vi "Edit_Server_Channel.vi"(5 "Mode":T1(ring)) -> ()   [LabVIEW 2021]
uses:
  Sub VIs/ADAM Controls/Ch_description_ADAM.ctl
  Sub VIs/ADAM Controls/Module_type_ADAM.ctl
  Sub VIs/ADAM Controls/Function_ADAM.ctl
  Sub VIs/ADAM Controls/Channel_State.ctl
  Sub VIs/ADAM Controls/Calib_type_ADAM.ctl
  Sub VIs/ADAM Controls/Address.ctl
  Sub VIs/ADAM Controls/Channel_names.ctl
panel:
  out "Message":string
  in  "Value":dbl
  out "String":string
  out "Help":string
  in  "Search String":string
  in  "Channel Names":i32(listbox)
  in  "Ch Description":T2={"Ch Name"="", "Type"="", "Function"=enum."Analogue Input", "Ch State"=enum."On", "Calibration type"="", "A"=0.0, "B"=0.0, "C"=0.0, "D"=0.0, "Comments"="", "Address"={"Main"=0, "Ch."=0, "Sub"=0, "Port Name"=""}, "String"="", "Duty"=65535} {"Duty" format="%016b"; "D" format="%#_5g"; "C" format="%#_5g"; "B" format="%#_5g"; "A" format="%#_5g"}
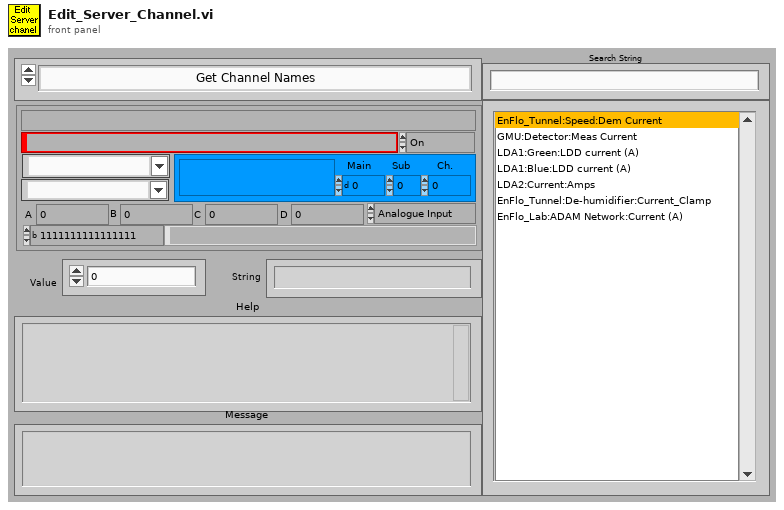
[diagram p1: front panel]
types:
  T1 = enum16{"Get Channel Names", "Get Current Value", "Update Channel Value", "Update Channel Description"}
  T2 = typedef "Ch_description_ADAM.ctl" = cluster{"Ch Name":string, "Type":T3, "Function":T4, "Ch State":T5, "Calibration type":T6, "A":dbl, "B":dbl, "C":dbl, "D":dbl, "Comments":string, "Address":T7, "String":string, "Duty":u16}
  T3 = typedef "Module_type_ADAM.ctl" = string
  T4 = typedef "Function_ADAM.ctl" = enum16{"Analogue Input", "Digital Input", "Event counter", "Event rate", "Analogue Output", "Digital Output", "Relay Output"}
  T5 = typedef "Channel_State.ctl" = enum16{"On", "Off", "Always On", "Always Off"}
  T6 = typedef "Calib_type_ADAM.ctl" = string
  T7 = typedef "Address.ctl" = cluster{"Main":i32, "Ch.":i32, "Sub":i32, "Port Name":string}
  T8 = typedef "Channel_names.ctl" = enum16{"Active Only", "Active + Off", "All Channels"}
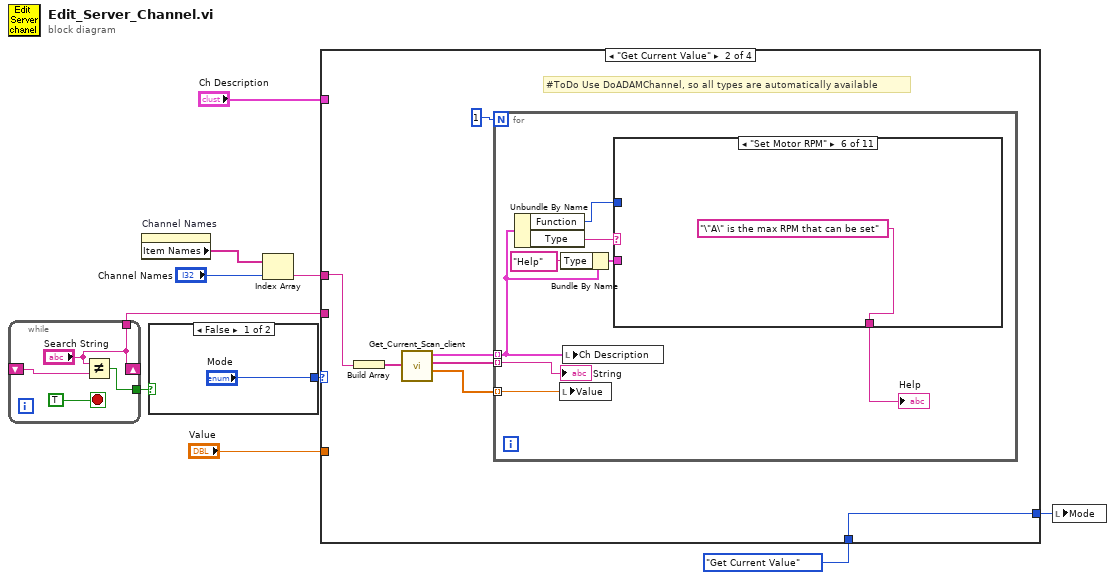
[diagram p0: block diagram]
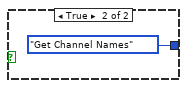
[diagram p2: hidden frame]
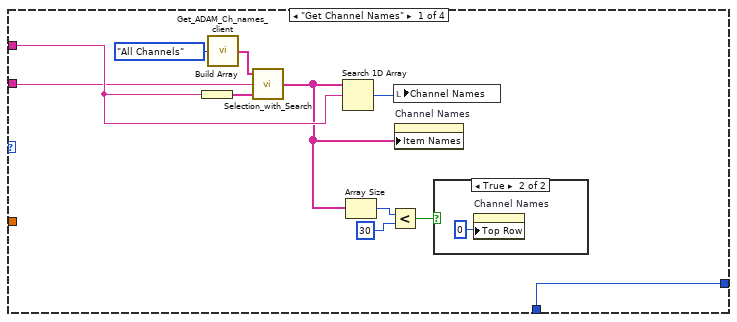
[diagram p3: hidden frame]
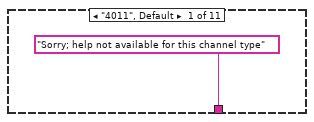
[diagram p5: hidden frame]
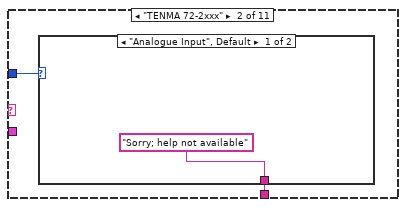
[diagram p6: hidden frame]
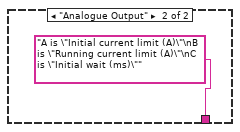
[diagram p7: hidden frame]
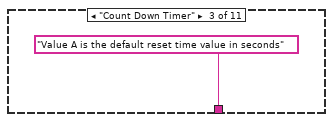
[diagram p8: hidden frame]
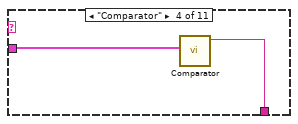
[diagram p9: hidden frame]
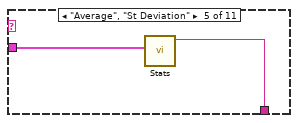
[diagram p10: hidden frame]
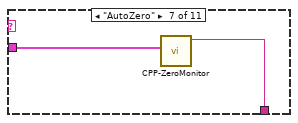
[diagram p11: hidden frame]
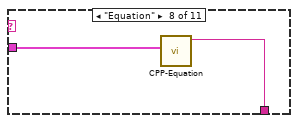
[diagram p12: hidden frame]
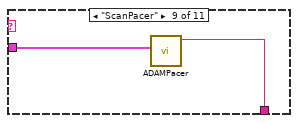
[diagram p13: hidden frame]
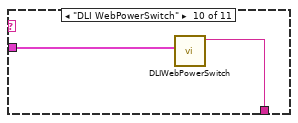
[diagram p14: hidden frame]
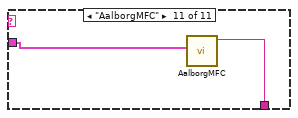
[diagram p15: hidden frame]
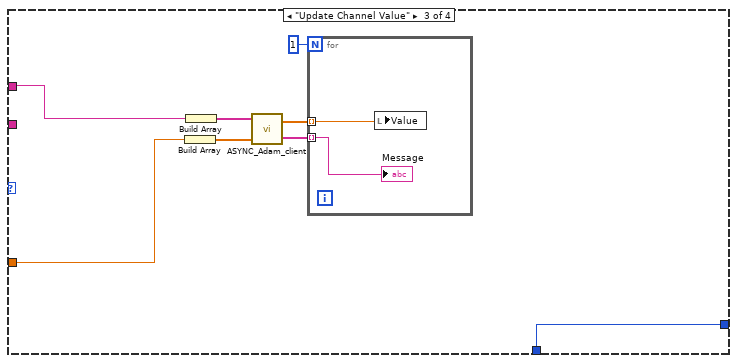
[diagram p16: hidden frame]
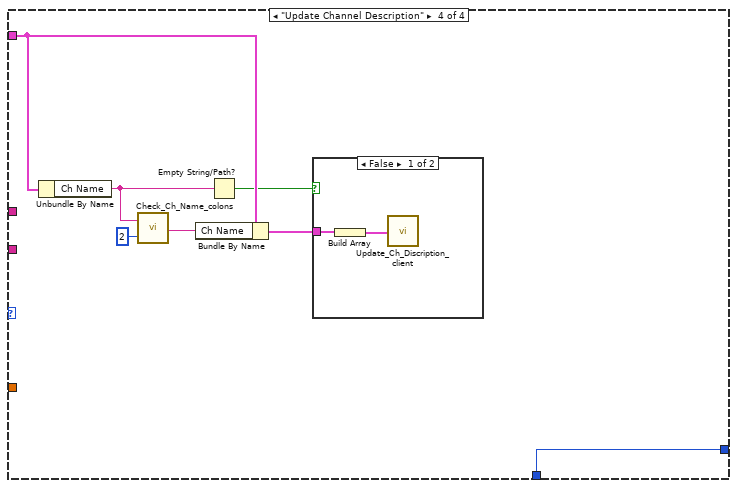
[diagram p17: hidden frame]
diagram:
  n1 = while {
    shift-right: ["Search String"] -> _
    shift-left: _ -> [w14]
    tunnel: [w13] -> w3
    tunnel: ["Search String"] -> w2
    stop <- TRUE stop-if-true
    n2 = Not Equal?(x="Search String", y=w14) -> (x != y?=w13:bool)
  }
  n3 = property on="Channel Names" class="LstBox (strict)"() -> ("Item Names"=w8:string[])  [unwired: 2 in, 2 out]
  n4 = case shown="False" w3 {
    tunnel: ["Mode" T1."Get Channel Names" ("Mode")] -> w10
    frame False {
    }
    frame True {
    }
  }
  n5 = Index Array(array=w8, index="Channel Names") -> (element=w7:string)
  n6 = case shown="\"Get Current Value\"" w10 {
    tunnel: w7 -> [w23 w34 w72 _]
    tunnel: "Value" -> [_ _ w69 _]
    tunnel: "Ch Description" -> [_ _ _ w80]
    tunnel: T1."Get Current Value" ("Mode") -> [w26 w29 w65 w81]
    tunnel: [w26 w29 w65 w81] -> w4
    tunnel: w2 -> [w21 _ _ _]
    frame "Get Channel Names" {
      n7 = Build Array(w23) -> (w24:string[])
      n8 = call "Get_ADAM_Ch_names_client.vi"("Channel names set"=Channel_names."All Channels") -> ("Ch names"=w25:string[])
      n9 = call "Selection_with_Search.vi"("Selected Channel Names"=w24, "Search String"=w21, "All Channel Names"=w25) -> ("Item Names"=w20:string[])
      n10 = Search 1D Array(1D array=w20, element=w23) -> (index of element=w22:i32)  [unwired: 1 out]
      n11 = Array Size(array=w20) -> (size(s)=w19:i32)
      n12 = Less?(x=w19, y=30) -> (x < y?=w17:bool)
      n13 = local write "Channel Names"(w22) -> ()
      n14 = property on="Channel Names" class="LstBox (strict)"("Item Names"=w20) -> ()  [unwired: 2 in, 2 out]
      n15 = case shown="True" w17 {
        frame False {
        }
        frame True {
          n16 = property on="Channel Names" class="LstBox (strict)"("Top Row"=0) -> ()  [unwired: 2 in, 2 out]
        }
      }
    }
    frame "Get Current Value" {
      # "#ToDo Use DoADAMChannel, so all types are automatically available"
      n17 = Build Array(w34) -> (w35:string[])
      n18 = call "Get_Current_Scan_client.vi"("multipleChannels"=w35) -> ("Ch Description Array"=w32:T2[], "String values"=w31:string[], "Numerical Values"=w30:dbl[])  [unwired: 1 in, 1 out]
      n19 = for {
        N: 1 -> [_]
        tunnel: w32 -> [w41] mode=indexing
        tunnel: w31 -> [w38] mode=indexing
        tunnel: w30 -> [w37] mode=indexing
        n20 = Unbundle By Name(w41) -> ("Function"=w36:T4, "Type"=w43:T3)
        n21 = local write "Value"(w37) -> ()
        n22 = Bundle By Name(cluster=w41, "Type"=T3 "Help") -> (w40:T2)
        n23 = local write "Ch Description"(w41) -> ()
        n24 = case shown="\"Set Motor RPM\"" w43 {
          tunnel: ["Sorry; help not available for this channel type" w45 "Value A is the default reset time value in seconds" w51 w52 "\"A\" is the max RPM that can be set" w55 w57 w59 w61 w63] -> w39
          tunnel: w40 -> [_ _ _ w50 w53 _ w56 w58 w60 w62 w64]
          tunnel: w36 -> [_ w46 _ _ _ _ _ _ _ _ _]
          frame "4011", Default {
          }
          frame "TENMA 72-2xxx" {
            n25 = case shown="\"Analogue Input\", Default" w46 {
              tunnel: ["Sorry; help not available" "A is \"Initial current limit (A)\"\nB is \"Running current limit (A)\"\nC is \"Initial wait (ms)\""] -> w45
              frame "Analogue Input", Default {
              }
              frame "Analogue Output" {
              }
            }
          }
          frame "Count Down Timer" {
          }
          frame "Comparator" {
            n26 = call "Comparator.vi"("Ch Description"=w50) -> ("HelpText"=w51:string)  [unwired: 6 in, 2 out]
          }
          frame "Average", "St Deviation" {
            n27 = call "Stats.vi"("Ch Description"=w53) -> ("HelpText"=w52:string)  [unwired: 6 in, 2 out]
          }
          frame "Set Motor RPM" {
          }
          frame "AutoZero" {
            n28 = call "CPP-ZeroMonitor.vi"("Ch Description"=w56) -> ("HelpText"=w55:string)  [unwired: 6 in, 2 out]
          }
          frame "Equation" {
            n29 = call "CPP-Equation.vi"("Ch Description"=w58) -> ("HelpText"=w57:string)  [unwired: 6 in, 2 out]
          }
          frame "ScanPacer" {
            n30 = call "ADAMPacer.vi"("Ch Description"=w60) -> ("HelpText"=w59:string)  [unwired: 6 in, 2 out]
          }
          frame "DLI WebPowerSwitch" {
            n31 = call "DLIWebPowerSwitch.vi"("Ch Description"=w62) -> ("HelpText"=w61:string)  [unwired: 6 in, 2 out]
          }
          frame "AalborgMFC" {
            n32 = call "AalborgMFC.vi"("Ch Description"=w64) -> ("HelpText"=w63:string)  [unwired: 6 in, 2 out]
          }
        }
        "Help" <- w39
        "String" <- w38
      }
    }
    frame "Update Channel Value" {
      n33 = Build Array(w69) -> (w70:dbl[])
      n34 = Build Array(w72) -> (w71:string[])
      n35 = call "ASYNC_Adam_client.vi"("Values"=w70, "Channel Names"=w71) -> ("Scan Comments"=w66:string[], "Calibrated Units"=w67:dbl[])  [unwired: 1 in]
      n36 = for {
        N: 1 -> [_]
        tunnel: w67 -> [w74] mode=indexing
        tunnel: w66 -> [w73] mode=indexing
        n37 = local write "Value"(w74) -> ()
        "Message" <- w73
      }
    }
    frame "Update Channel Description" {
      n38 = Unbundle By Name(w80) -> ("Ch Name"=w79:string)
      n39 = call "Check_Ch_Name_colons.vi"("No of Colons"=2, "Ch Name in"=w79) -> ("Ch Name out"=w77:string)
      n40 = Bundle By Name(cluster=w80, "Ch Name"=w77) -> (w76:T2)
      n41 = Empty String/Path?(string/path=w79) -> (empty?=w75:bool)
      n42 = case shown="False" w75 {
        tunnel: w76 -> [w82 _]
        frame False {
          n43 = Build Array(w82) -> (w83:T2[])
          n44 = call "Update_Ch_Discription_client.vi"("Channels to update In"=w83) -> ()  [unwired: 1 out]
        }
        frame True {
        }
      }
    }
  }
  n45 = local write "Mode"(w4) -> ()
